vi "Create DSF UDP Loopback Configuration Files.vi"() -> ()   [LabVIEW 2017]
uses:
  DSF Core.lvlibp/Classes/Configuration/Configuration Session.lvclass
  DSF Core.lvlibp/Typedefs/DSF Timing Info.ctl
  DSF Core.lvlibp
  DSF Core.lvlibp/Typedefs/DSF Settings Info.ctl
  DSF Core.lvlibp/Typedefs/DSF Engine Plugin Thread Configuration.ctl
  DSF Core.lvlibp/Typedefs/DSF Direction.ctl
  DSF Core.lvlibp/Typedefs/DSF Byte Order.ctl
  DSF Core.lvlibp/Typedefs/DSF Data Type.ctl
  DSF Core.lvlibp/Typedefs/DSF Engine Channel Configuration.ctl
  DSF Core.lvlibp/Typedefs/DSF Engine Transfer Configuration.ctl
  DSF Core.lvlibp/Typedefs/DSF Timeout Behavior.ctl
  DSF Core.lvlibp/Typedefs/DSF Engine Transfer Group Configuration.ctl
  DSF Core.lvlibp/Typedefs/DSF Engine Plugin Configuration.ctl
  DSF Core.lvlibp/Typedefs/DSF Engine Framework Configuration.ctl
panel:
  in  "Tx Ports":u16[](array[numeric])
  in  "Rx Ports":u16[](array[numeric])
  out "Framework Configuration":T1
  in  "channels data type":T11=enum."SGL"
  in  "channel count per transfer":u64=1000
  in  "Destination IP Address":string="localhost"
  in  "Source IP Address":string="localhost"
  in  "Local Ports":u16[](array[numeric])
  out "error out":errorcluster
  in  "error in (no error)":errorcluster
  in  "Output Folder":path
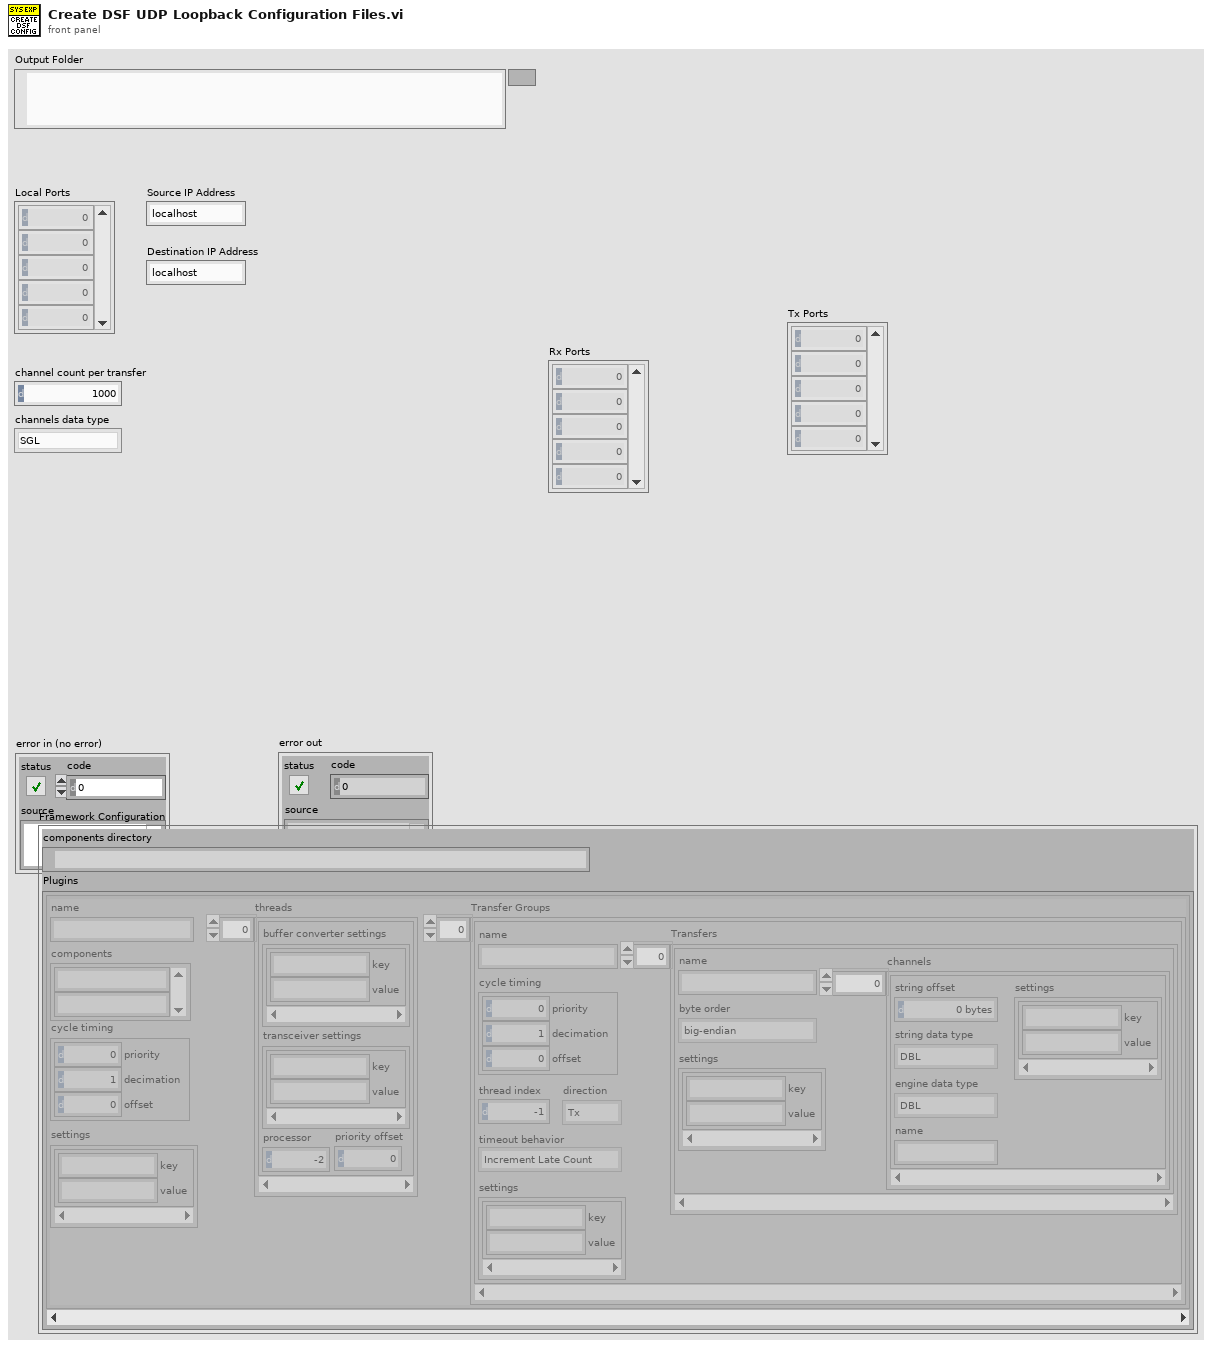
[diagram p1: front panel]
types:
  T1 = typedef "DSF Core.lvlibp/DSF Engine Framework Configuration.ctl" = cluster{"components directory":path, "Plugins":T2[]}
  T2 = typedef "DSF Core.lvlibp/DSF Engine Plugin Configuration.ctl" = cluster{"name":string, "components":string[], "cycle timing":T3, "threads":T4[], "Transfer Groups":T6[], "settings":T5}
  T3 = typedef "DSF Core.lvlibp/DSF Timing Info.ctl" = cluster{"priority":u64, "decimation":u64, "offset":u64}
  T4 = typedef "DSF Core.lvlibp/DSF Engine Plugin Thread Configuration.ctl" = cluster{"buffer converter settings":T5, "transceiver settings":T5, "processor":i32, "priority offset":i16}
  T5 = typedef "DSF Core.lvlibp/DSF Settings Info.ctl" = cluster{"key":string, "value":string}[]
  T6 = typedef "DSF Core.lvlibp/DSF Engine Transfer Group Configuration.ctl" = cluster{"name":string, "direction":T7, "cycle timing":T3, "thread index":i32, "settings":T5, "Transfers":T8[], "timeout behavior":T12}
  T7 = typedef "DSF Core.lvlibp/DSF Direction.ctl" = enum8{"Tx", "Rx"}
  T8 = typedef "DSF Core.lvlibp/DSF Engine Transfer Configuration.ctl" = cluster{"name":string, "byte order":T9, "settings":T5, "channels":T10[]}
  T9 = typedef "DSF Core.lvlibp/DSF Byte Order.ctl" = enum8{"big-endian", "little-endian"}
  T10 = typedef "DSF Core.lvlibp/DSF Engine Channel Configuration.ctl" = cluster{"string offset":u64, "string data type":T11, "engine data type":T11, "name":string, "settings":T5}
  T11 = typedef "DSF Core.lvlibp/DSF Data Type.ctl" = enum8{"Bool", "SGL", "DBL", "I8", "I16", "I32", "I64", "U8", "U16", "U32", "U64"}
  T12 = typedef "DSF Core.lvlibp/DSF Timeout Behavior.ctl" = enum8{"Increment Late Count", "Throw Error"}
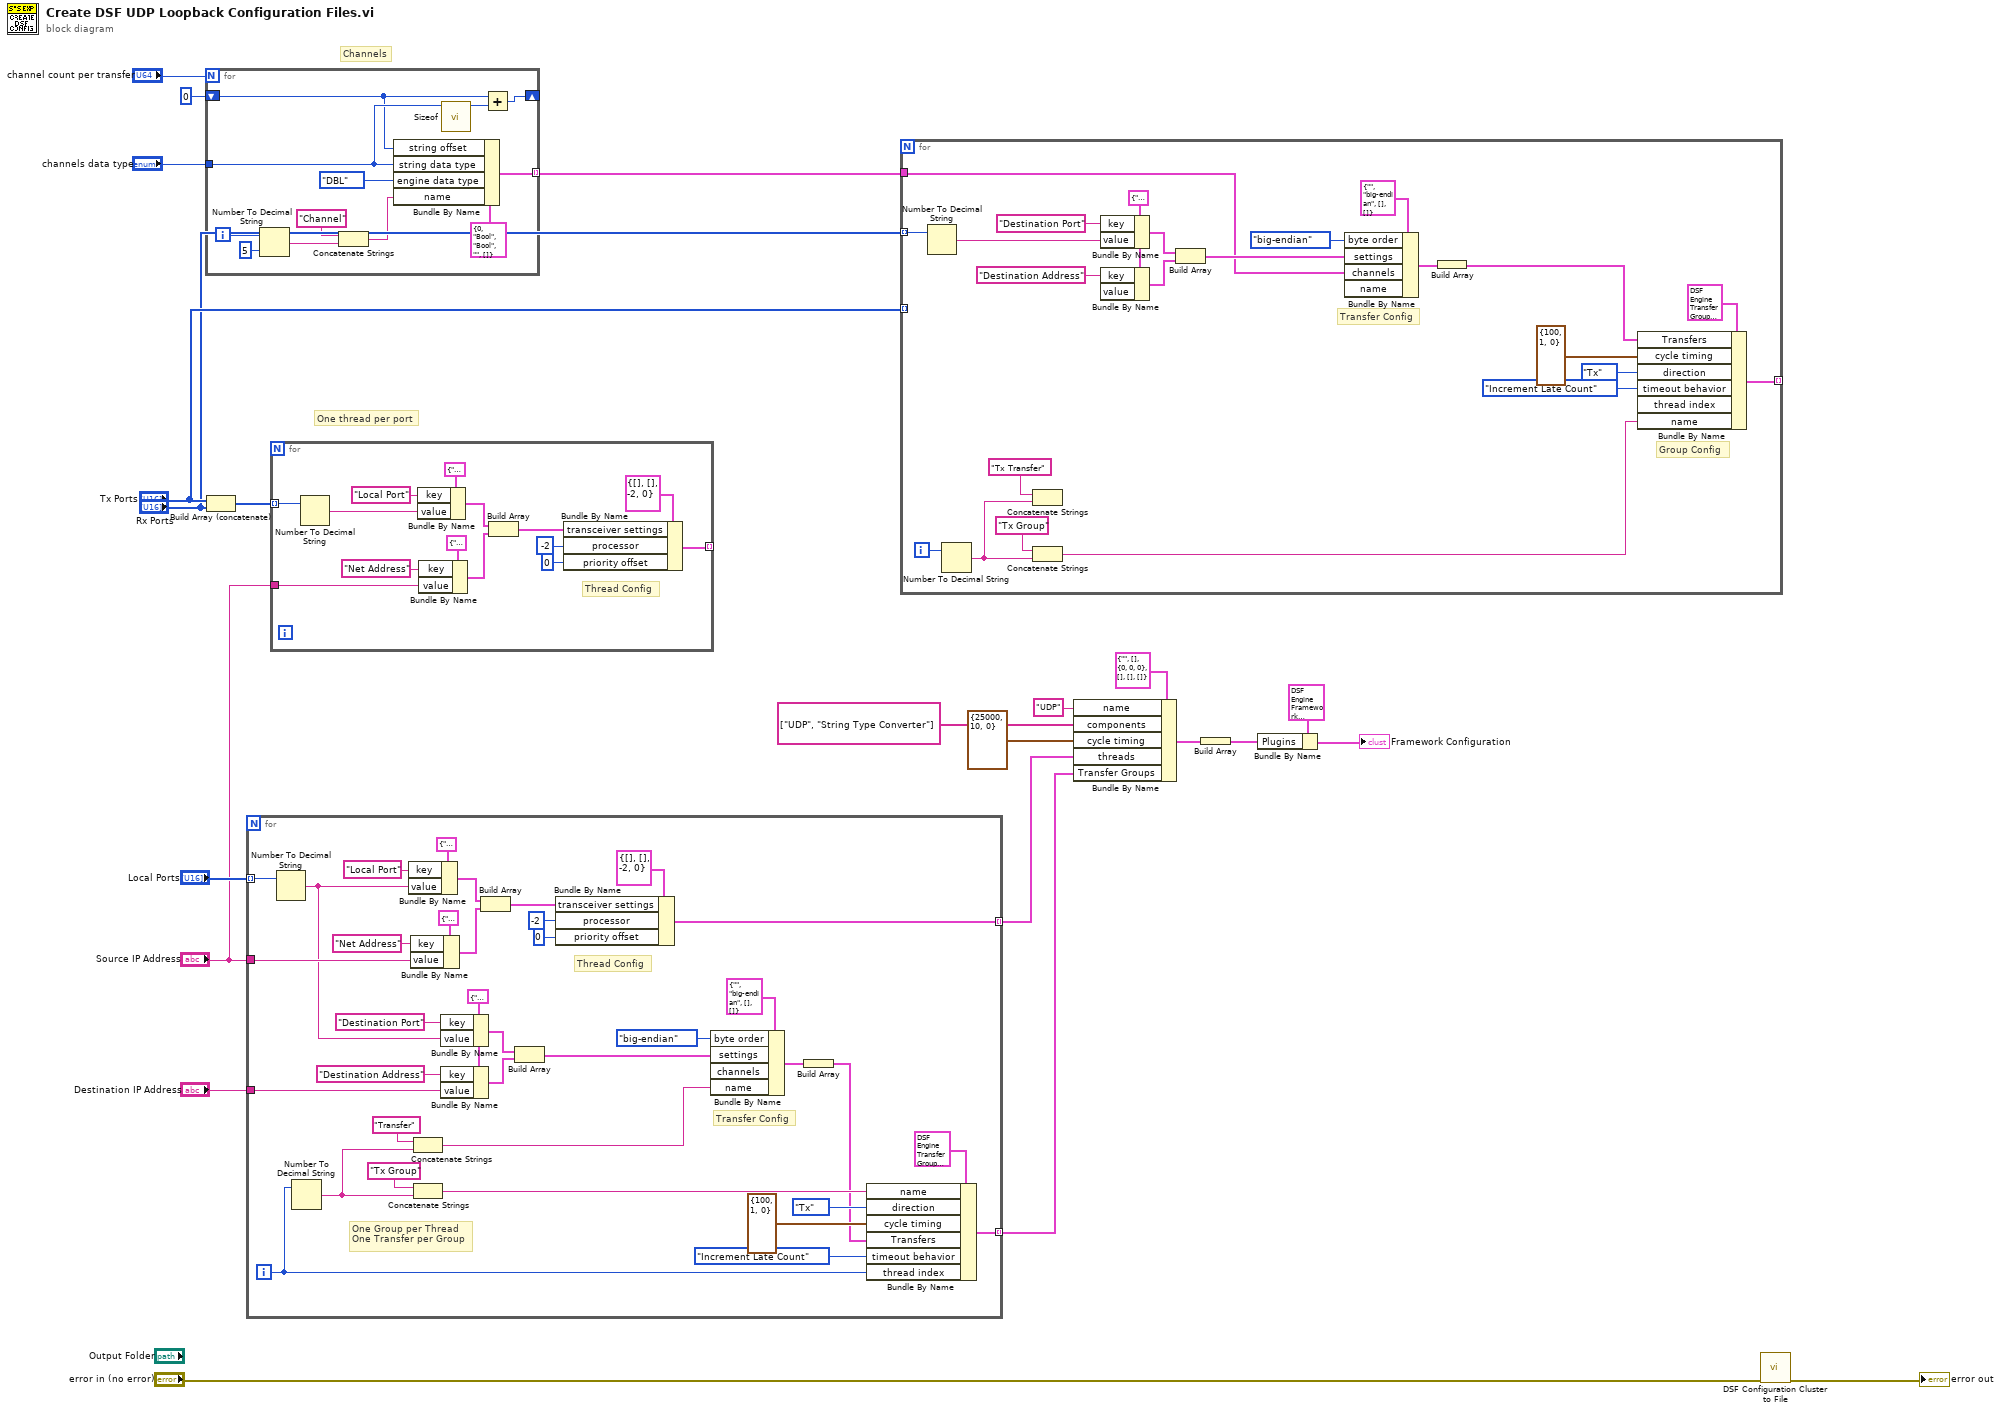
[diagram p0: block diagram]
diagram:
  # "Channels"
  # "One thread per port"
  n1 = for {
    N: "channel count per transfer" -> [_]
    tunnel: "channels data type" -> [w32]
    shift-right: [w24] -> _
    shift-left: u64 0 ("string offset") -> [w25]
    tunnel: [w23] -> w2 mode=indexing
    i -> [w30]
    n2 = Number To Decimal String(number=w30, width (-)=i16 5) -> (decimal integer string=w28:string)
    n3 = Concatenate Strings("Channel" ("name"), w28) -> (w27:string)
    n4 = Bundle By Name(cluster=T10 {"string offset"=0, "string data type"=enum."Bool", "engine data type"=enum."Bool", "name"="", "settings"=[]} ("channel configuration"), "string offset"=w25, "string data type"=w32, "engine data type"=DSF_Data_Type."DBL", "name"=w27) -> (w23:T10)
    n5 = call "Sizeof.vi"("data type"=w32) -> ("size in bytes"=w26:u64)  [unwired: 9 in, 1 out]
    n6 = Add(x=w25, y=w26) -> (x+y=w24:u64)
  }
  n7 = Build Array (concatenate)("Tx Ports", "Rx Ports") -> (w8:u16[])
  n8 = for {
    tunnel: "Local Ports" -> [w60] mode=indexing
    tunnel: [w59] -> w14 mode=indexing
    tunnel: "Source IP Address" -> [w58]
    tunnel: [w49] -> w13 mode=indexing
    tunnel: "Destination IP Address" -> [w40]
    i -> [w52]
    w46 = cluster{"key":string, "value":string} {"key"="Local Port", "value"="50000"} ("setting")
    # "Group Config"
    # "Transfer Config"
    # "One Group per Thread\nOne Transfer per Group"
    # "Thread Config"
    n9 = Number To Decimal String(number=w60) -> (decimal integer string=w41:string)  [unwired: 1 in]
    n10 = Number To Decimal String(number=w52) -> (decimal integer string=w35:string)  [unwired: 1 in]
    n11 = Bundle By Name(cluster=cluster{"key":string, "value":string} {"key"="Local Port", "value"="50000"} ("setting"), "key"="Local Port", "value"=w41) -> (w63:cluster{"key":string, "value":string})
    n12 = Bundle By Name(cluster=cluster{"key":string, "value":string} {"key"="Local Port", "value"="50000"} ("setting"), "key"="Net Address", "value"=w58) -> (w62:cluster{"key":string, "value":string})
    n13 = Concatenate Strings("Transfer" ("name"), w35) -> (w36:string)
    n14 = Concatenate Strings("Tx Group" ("name"), w35) -> (w45:string)
    n15 = Bundle By Name(cluster=w46, "key"="Destination Port", "value"=w41) -> (w42:cluster{"key":string, "value":string})
    n16 = Bundle By Name(cluster=w46, "key"="Destination Address", "value"=w40) -> (w43:cluster{"key":string, "value":string})
    n17 = Build Array(w63, w62) -> (w61:cluster{"key":string, "value":string}[])
    n18 = Build Array(w42, w43) -> (w39:cluster{"key":string, "value":string}[])
    n19 = Bundle By Name(cluster=T4 {"buffer converter settings"=[], "transceiver settings"=[], "processor"=-2, "priority offset"=0} ("threads"), "transceiver settings"=w61, "processor"=-2, "priority offset"=i16 0) -> (w59:T4)
    n20 = Bundle By Name(cluster=T8 {"name"="", "byte order"=enum."big-endian", "settings"=[], "channels"=[]} ("Transfer Configuration"), "byte order"=DSF_Byte_Order."big-endian", "settings"=w39, "name"=w36) -> (w38:T8)  [unwired: 1 in]
    n21 = Build Array(w38) -> (w37:T8[])
    n22 = Bundle By Name(cluster=T6 {"name"="", "direction"=enum."Tx", "cycle timing"={"priority"=0, "decimation"=0, "offset"=0}, "thread index"=0, "settings"=[], "Transfers"=[], "timeout behavior"=enum."Increment Late Count"} ("Transfer Group Configuration"), "name"=w45, "direction"=DSF_Direction."Tx", "cycle timing"=T3 {"priority"=100, "decimation"=1, "offset"=0}, "Transfers"=w37, "timeout behavior"=DSF_Timeout_Behavior."Increment Late Count", "thread index"=w52) -> (w49:T6)
  }
  n23 = for {
    tunnel: w8 -> [w74] mode=indexing
    tunnel: [w73] -> _ mode=indexing
    tunnel: "Source IP Address" -> [w72]
    # "Thread Config"
    n24 = Number To Decimal String(number=w74) -> (decimal integer string=w71:string)  [unwired: 1 in]
    n25 = Bundle By Name(cluster=cluster{"key":string, "value":string} {"key"="Local Port", "value"="50000"} ("setting"), "key"="Local Port", "value"=w71) -> (w77:cluster{"key":string, "value":string})
    n26 = Bundle By Name(cluster=cluster{"key":string, "value":string} {"key"="Local Port", "value"="50000"} ("setting"), "key"="Net Address", "value"=w72) -> (w76:cluster{"key":string, "value":string})
    n27 = Build Array(w77, w76) -> (w75:cluster{"key":string, "value":string}[])
    n28 = Bundle By Name(cluster=T4 {"buffer converter settings"=[], "transceiver settings"=[], "processor"=-2, "priority offset"=0} ("threads"), "transceiver settings"=w75, "processor"=-2, "priority offset"=i16 0) -> (w73:T4)
  }
  n29 = for {
    tunnel: "Tx Ports" -> [_] mode=indexing
    tunnel: [w100] -> _ mode=indexing
    tunnel: w2 -> [w90]
    tunnel: "Rx Ports" -> [w86] mode=indexing
    i -> [w104]
    w93 = cluster{"key":string, "value":string} {"key"="Local Port", "value"="50000"} ("setting")
    # "Transfer Config"
    # "Group Config"
    n30 = Number To Decimal String(number=w86) -> (decimal integer string=w85:string)  [unwired: 1 in]
    n31 = Number To Decimal String(number=w104) -> (decimal integer string=w88:string)  [unwired: 1 in]
    n32 = Concatenate Strings("Tx Transfer" ("name"), w88) -> ()  [unwired: 1 out]
    n33 = Concatenate Strings("Tx Group" ("name"), w88) -> (w103:string)
    n34 = Bundle By Name(cluster=w93, "key"="Destination Port", "value"=w85) -> (w97:cluster{"key":string, "value":string})
    n35 = Bundle By Name(cluster=w93, "key"="Destination Address") -> (w96:cluster{"key":string, "value":string})  [unwired: 1 in]
    n36 = Build Array(w97, w96) -> (w98:cluster{"key":string, "value":string}[])
    n37 = Bundle By Name(cluster=T8 {"name"="", "byte order"=enum."big-endian", "settings"=[], "channels"=[]} ("Transfer Configuration"), "byte order"=DSF_Byte_Order."big-endian", "settings"=w98, "channels"=w90) -> (w99:T8)  [unwired: 1 in]
    n38 = Build Array(w99) -> (w87:T8[])
    n39 = Bundle By Name(cluster=T6 {"name"="", "direction"=enum."Tx", "cycle timing"={"priority"=0, "decimation"=0, "offset"=0}, "thread index"=0, "settings"=[], "Transfers"=[], "timeout behavior"=enum."Increment Late Count"} ("Transfer Group Configuration"), "Transfers"=w87, "cycle timing"=T3 {"priority"=100, "decimation"=1, "offset"=0}, "direction"=DSF_Direction."Tx", "timeout behavior"=DSF_Timeout_Behavior."Increment Late Count", "name"=w103) -> (w100:T6)  [unwired: 1 in]
  }
  n40 = Bundle By Name(cluster=T2 {"name"="", "components"=[], "cycle timing"={"priority"=0, "decimation"=0, "offset"=0}, "threads"=[], "Transfer Groups"=[], "settings"=[]} ("Plugin Configuration"), "name"="UDP", "components"=string[] ["UDP", "String Type Converter"], "cycle timing"=T3 {"priority"=25000, "decimation"=10, "offset"=0}, "threads"=w14, "Transfer Groups"=w13) -> (w12:T2)
  n41 = Build Array(w12) -> (w11:T2[])
  n42 = Bundle By Name(cluster=T1 {"components directory"=path "", "Plugins"=[{"name"="UDP", "components"=["UDP", "String Type Converter"], "cycle timing"={"priority"=25000, "decimation"=10, "offset"=0}, "threads"=[], "Transfer Groups"=[], "settings"=[]}]} ("framework configuration"), "Plugins"=w11) -> (→"Framework Configuration":T1)
  n43 = call "DSF Configuration Cluster to File.vi"("error in (no error)"="error in (no error)") -> ("error out"=→"error out":errorcluster)  [unwired: 9 in, 1 out]
